vi "update_reactor_cluster.vi"(6 "THROW OUT EVENTS":i32=500, 8 "error in":errorcluster, 9 "NEW DATA":sgl[][](array[numeric]), 10 "Reactor to update (INDEX)":i32, 11 "REACTORS":T1) -> (0 "error out":errorcluster, 3 "UPDATED REACTORS":T1)   [LabVIEW 2013]
uses:
  type_defs/reactors.ctl
  type_defs/reactor.ctl
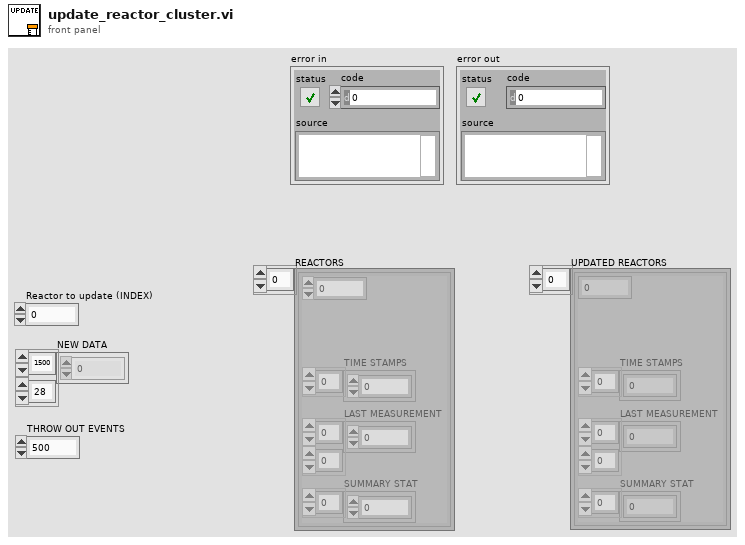
[diagram p1: front panel]
types:
  T1 = typedef "reactors.ctl" = cluster{i32, "TIME STAMPS":dbl[], "LAST MEASUREMENT":T2[][], "SUMMARY STAT":dbl[]}[]
  T2 = typedef "reactor.ctl" = dbl
  T3 = cluster{i32, "TIME STAMPS":dbl[], "LAST MEASUREMENT":T2[][], "SUMMARY STAT":dbl[]}
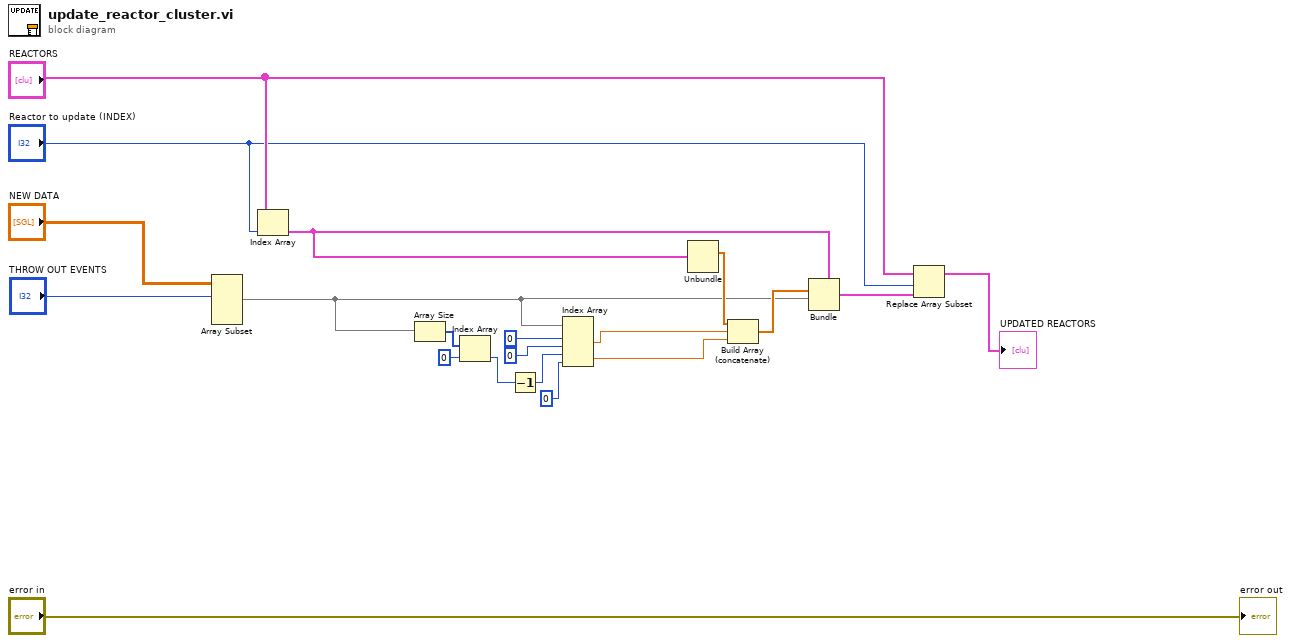
[diagram p0: block diagram]
diagram:
  n1 = Array Subset(array="NEW DATA", index (row)="THROW OUT EVENTS") -> (w1:sgl[][])  [unwired: 3 in]
  n2 = Index Array(array="REACTORS", index="Reactor to update (INDEX)") -> (element=w14:T3)
  n3 = Array Size(array=w1) -> (size(s)=w13:i32[])
  n4 = Index Array(array=w13, index=0) -> (element=w9:i32)
  n5 = Decrement(x=w9) -> (x-1=w7:i32)
  n6 = Index Array(array=w1, index (row) #1=0 ("disabled index (row)"), index (col) #1=0 ("disabled index (col)"), index (row) #2=w7, index (col) #2=0 ("index (row)")) -> (element #1=w4:sgl, element #2=w5:sgl)
  n7 = Unbundle(w14) -> ("TIME STAMPS"=w3:dbl[])  [unwired: 3 out]
  n8 = Build Array (concatenate)(w3, w4, w5) -> (w2:dbl[])
  n9 = Bundle(cluster=w14, "TIME STAMPS"=w2, "LAST MEASUREMENT"=w1) -> (w16:T3)  [unwired: 2 in]
  n10 = Replace Array Subset(array="REACTORS", new element=w16, index="Reactor to update (INDEX)") -> (→"UPDATED REACTORS":T1)
  "error out" <- "error in"
